vi "p2.vi"() -> ()   [LabVIEW 2025, in "d1.lvlib"]
uses:
  d1.lvlib
  AOC/AOC.lvlib
panel:
  in  "Example":string="L50\nL50"
  in  "Example?":bool
  out "Answer":i64=55607
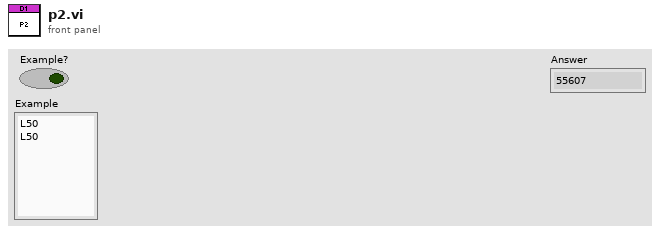
[diagram p1: front panel]
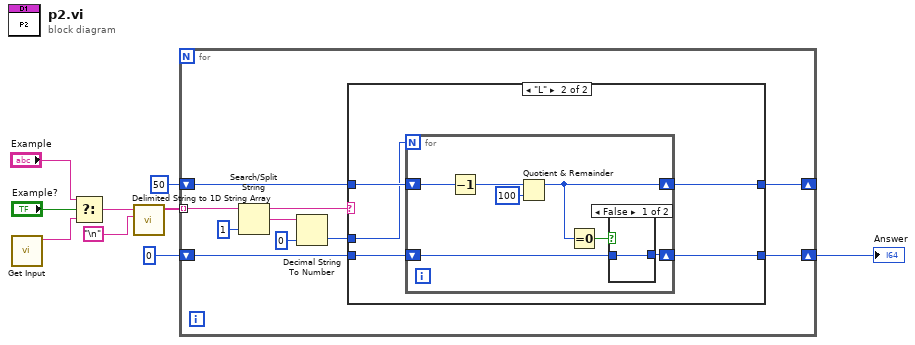
[diagram p0: block diagram]
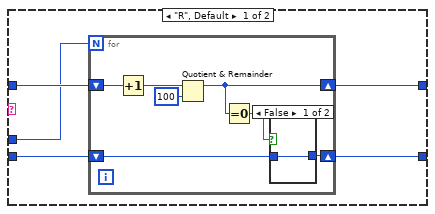
[diagram p2: hidden frame]
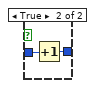
[diagram p3: hidden frame]
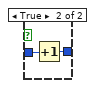
[diagram p4: hidden frame]
diagram:
  n1 = call "Get Input.vi"() -> ("Input"=w8:string)  [unwired: 11 in]
  n2 = Select(t="Example", s="Example?", f=w8) -> (s? t:f=w6:string)
  n3 = call <vilib>:"Delimited String to 1D String Array.vi"("delimiter"="\n", "delimited string"=w6) -> ("string array"=w4:string[])  [unwired: 9 in]
  n4 = for {
    tunnel: w4 -> [w19] mode=indexing
    shift-right: [w10] -> _
    shift-left: i64 50 ("Answer") -> [w17]
    shift-right: [w11] -> w1
    shift-left: i64 0 ("Answer") -> [w12]
    n5 = Search/Split String(string=w19, offset (0)=1) -> (substring before match=w16:string, match + rest of string=w15:string)  [unwired: 1 in, 1 out]
    n6 = Decimal String To Number(string=w15, default (0L)=i64 0 ("default (0 I32)")) -> (number=w14:i64)  [unwired: 1 in, 1 out]
    n7 = case shown="\"L\"" w16 {
      tunnel: w17 -> [w24 w39]
      tunnel: [w23 w38] -> w10
      tunnel: w14 -> [w22 w37]
      tunnel: w12 -> [w21 w36]
      tunnel: [w20 w35] -> w11
      frame "R", Default {
        n8 = for {
          N: w22 -> [_]
          shift-right: [w25] -> w23
          shift-left: w24 -> [w31]
          shift-right: [w28] -> w20
          shift-left: w21 -> [w29]
          n9 = Increment(x=w31) -> (x+1=w26:i64)
          n10 = Quotient & Remainder(x=w26, y=i64 100) -> (x-y*floor(x/y)=w25:i64)  [unwired: 1 out]
          n11 = Equal To 0?(x=w25) -> (x = 0?=w30:bool)
          n12 = case shown="False" w30 {
            tunnel: w29 -> [w32 w34]
            tunnel: [w32 w33] -> w28
            frame False {
            }
            frame True {
              n13 = Increment(x=w34) -> (x+1=w33:i64)
            }
          }
        }
      }
      frame "L" {
        n14 = for {
          N: w37 -> [_]
          shift-right: [w40] -> w38
          shift-left: w39 -> [w46]
          shift-right: [w43] -> w35
          shift-left: w36 -> [w44]
          n15 = Decrement(x=w46) -> (x-1=w41:i64)
          n16 = Quotient & Remainder(x=w41, y=i64 100) -> (x-y*floor(x/y)=w40:i64)  [unwired: 1 out]
          n17 = Equal To 0?(x=w40) -> (x = 0?=w45:bool)
          n18 = case shown="False" w45 {
            tunnel: w44 -> [w47 w49]
            tunnel: [w47 w48] -> w43
            frame False {
            }
            frame True {
              n19 = Increment(x=w49) -> (x+1=w48:i64)
            }
          }
        }
      }
    }
  }
  "Answer" <- w1
